vi "menu.vi"() -> ()   [LabVIEW 2017]
panel:
  in  "SALIR":bool
  in  "simulador de grafico":bool
  in  "simulador en tiempo real":bool
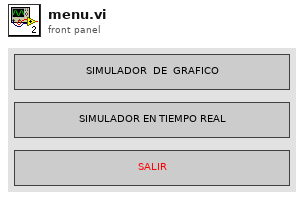
[diagram p1: front panel]
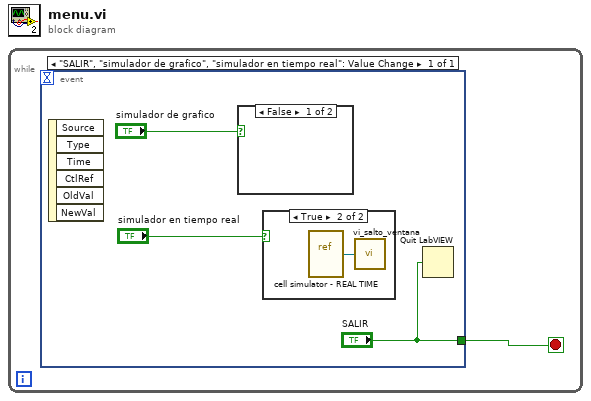
[diagram p0: block diagram]
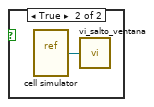
[diagram p2: hidden frame]
diagram:
  n1 = while {
    stop <- w1 stop-if-true
    n2 = event shown="[0] \"SALIR\", \"simulador de grafico\", \"simulador en tiempo real\": Value Change" {
      selector: _ -> [_]
      dyn-events: _ -> [_]
      timeout: _ -> [_]
      tunnel: ["SALIR"] -> w1
      event "SALIR", "simulador de grafico", "simulador en tiempo real": Value Change {
        n3 = event-data() -> ()  [unwired: 1 in, 6 out]
        n4 = case shown="False" "simulador de grafico" {
          frame False {
          }
          frame True {
            n5 = vi-ref "cell simulator.vi"() -> (w5:refnum<vi>)
            n6 = call "vi_salto_ventana.vi"("reference"=w5) -> ()
          }
        }
        n7 = case shown="True" "simulador en tiempo real" {
          frame False {
          }
          frame True {
            n8 = vi-ref "cell simulator - REAL TIME.vi"() -> (w6:refnum<vi>)
            n9 = call "vi_salto_ventana.vi"("reference"=w6) -> ()
          }
        }
        n10 = Quit LabVIEW(quit? (T)="SALIR") -> ()
      }
    }
  }
